vi "Registers.vi"(0 "register instruction":T6, 5 "config.resources":T4, 7 "sync.resources":T7, 9 "time.resources":T3) -> (4 "read completion out":T5, 14 "ready for input":bool)   [LabVIEW 2023]
uses:
  <instrlib>/niUSRPRIO/GPS/v1/FPGA/niUsrpRio GPS v1 FPGA.lvlib
  <instrlib>/niUsrpRio/Config/v1/FPGA/niUsrpRio Config v1 FPGA.lvlib
  <instrlib>/niUSRPRIO/Time/v1/FPGA/niUsrpRio Time v1 FPGA.lvlib
  <instrlib>/niUSRPRIO/Synchronization/v1/FPGA/niUsrpRio Synchronization v1 FPGA.lvlib
  <instrlib>/_niInstr/Register Bus/v1/FPGA/Private/Mux/Read Completion Mux (6 inputs).vi
  <instrlib>/niUSRPRIO/Synchronization/v1/FPGA/Private/Resources.ctl
  <instrlib>/_niInstr/Register Bus/v1/FPGA/Public/Register Instruction.ctl
  <instrlib>/niUSRPRIO/Time/v1/FPGA/Private/Future Event Resources.ctl
  <instrlib>/niUSRPRIO/Time/v1/FPGA/Private/Time Resources.ctl
  <instrlib>/_niInstr/Register Bus/v1/FPGA/Public/Read Completion.ctl
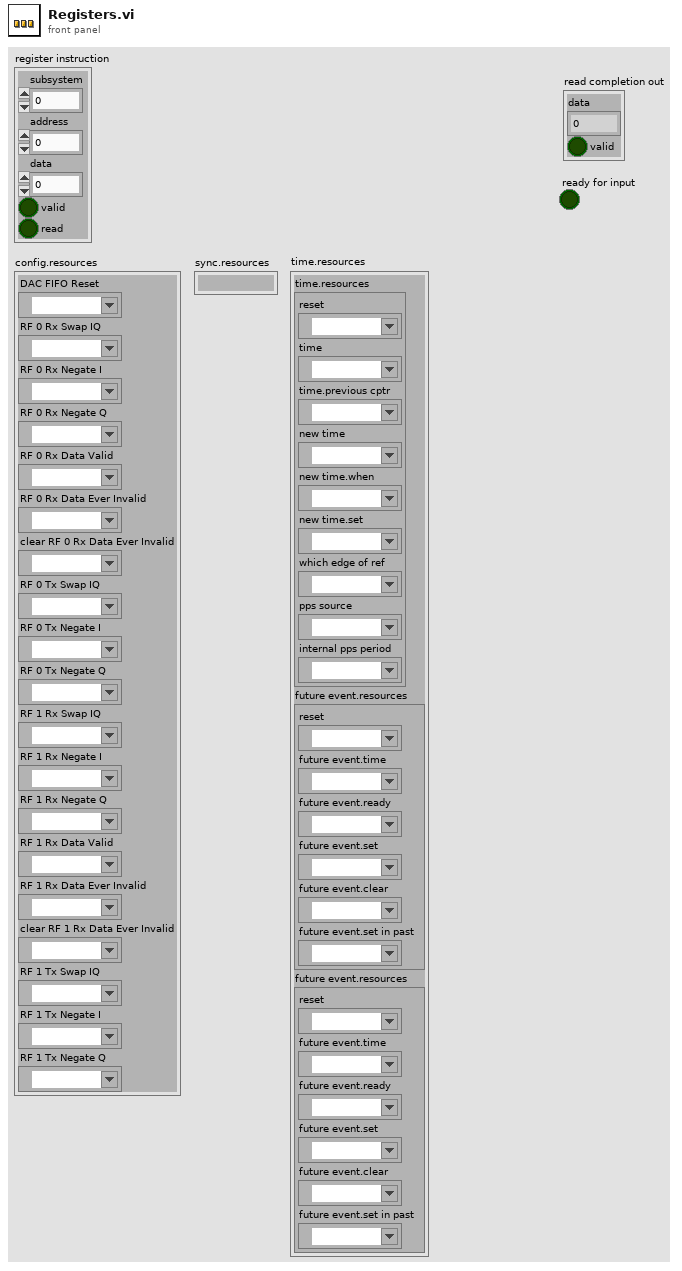
[diagram p1: front panel]
types:
  T1 = typedef "niUsrpRio Time v1 FPGA.lvlib/Time Resources.ctl" = cluster{"reset":refnum<k21>, "time":refnum<k21>, "time.previous cptr":refnum<k21>, "new time":refnum<k21>, "new time.when":refnum<k21>, "new time.set":refnum<k21>, "which edge of ref":refnum<k21>, "pps source":refnum<k21>, "internal pps period":refnum<k21>}
  T2 = typedef "niUsrpRio Time v1 FPGA.lvlib/Future Event Resources.ctl" = cluster{"reset":refnum<k21>, "future event.time":refnum<k21>, "future event.ready":refnum<k21>, "future event.set":refnum<k21>, "future event.clear":refnum<k21>, "future event.set in past":refnum<k21>}
  T3 = cluster{"time.resources":T1, "future event.resources":T2, "future event.resources":T2}
  T4 = cluster{"DAC FIFO Reset":refnum<k21>, "RF 0 Rx Swap IQ":refnum<k21>, "RF 0 Rx Negate I":refnum<k21>, "RF 0 Rx Negate Q":refnum<k21>, "RF 0 Rx Data Valid":refnum<k21>, "RF 0 Rx Data Ever Invalid":refnum<k21>, "clear RF 0 Rx Data Ever Invalid":refnum<k21>, "RF 0 Tx Swap IQ":refnum<k21>, "RF 0 Tx Negate I":refnum<k21>, "RF 0 Tx Negate Q":refnum<k21>, "RF 1 Rx Swap IQ":refnum<k21>, "RF 1 Rx Negate I":refnum<k21>, "RF 1 Rx Negate Q":refnum<k21>, "RF 1 Rx Data Valid":refnum<k21>, "RF 1 Rx Data Ever Invalid":refnum<k21>, "clear RF 1 Rx Data Ever Invalid":refnum<k21>, "RF 1 Tx Swap IQ":refnum<k21>, "RF 1 Tx Negate I":refnum<k21>, "RF 1 Tx Negate Q":refnum<k21>}
  T5 = typedef "niInstr Register Bus v1 FPGA.lvlib/Read Completion.ctl" = cluster{"data":u32, "valid":bool}
  T6 = typedef "niInstr Register Bus v1 FPGA.lvlib/Register Instruction.ctl" = cluster{"subsystem":u8, "address":u16, "data":u32, "valid":bool, "read":bool}
  T7 = typedef "niUsrpRio Synchronization v1 FPGA.lvlib/Resources.ctl" = cluster{"master":refnum<k21>, "meas.enable":refnum<k21>, "meas.ready":refnum<k21>, "meas.reset":refnum<k21>, "meas.arm":refnum<k21>, "meas.valid":refnum<k21>, "meas.value":refnum<k21>, "meas.oversample factor":refnum<k21>, "cptr":refnum<k21>, "cptr.adjust":refnum<k21>, "cptr.period":refnum<k21>}
  T8 = enum8{"rx.start trigger event", "tx.start trigger event"}
  T9 = cluster{"read completion":T5, "read completion":T5}
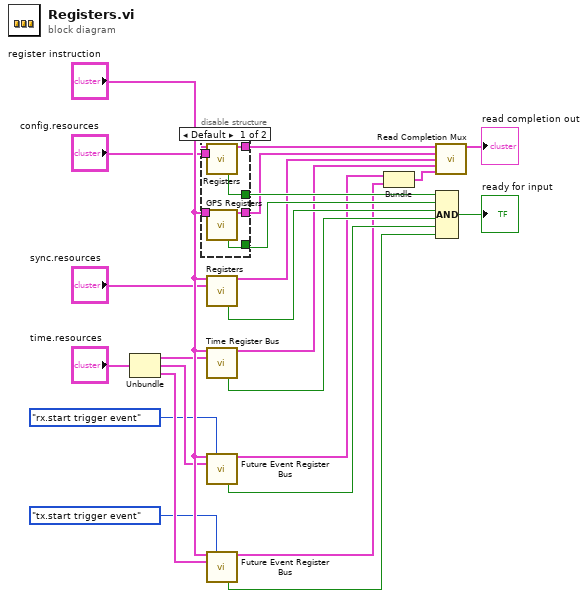
[diagram p0: block diagram]
diagram:
  n1 = Unbundle("time.resources") -> ("time.resources"=w5:T1, "future event.resources"=w4:T2, "future event.resources"=w3:T2)
  n2 = disable-structure shown="Default" {
    disable-tunnel: [w30 _] -> w20
    disable-tunnel: [w29 _] -> w19
    disable-tunnel: "register instruction" -> [w28 _]
    disable-tunnel: [w27 _] -> w11
    disable-tunnel: [w26 _] -> w10
    disable-tunnel: "config.resources" -> [w25 _]
    frame condition #0 (active) {
      n3 = call <instrlib>:"Registers.vi"("register instruction"=w28, "resources"=w25) -> ("read completion out"=w26:T5, "ready for input"=w29:bool)  [unwired: 12 in]
      n4 = call <instrlib>:"GPS Registers.vi"("register instruction"=w28) -> ("read completion"=w27:T5, "ready for input"=w30:bool)  [unwired: 13 in]
    }
    frame condition #1 {
    }
  }
  n5 = call <instrlib>:"Registers.vi"("register instruction"="register instruction", "sync.resources"="sync.resources") -> ("read completion"=w16:T5, "ready for input"=w21:bool)  [unwired: 12 in]
  n6 = call <instrlib>:"Time Register Bus.vi"("register instruction"="register instruction", "time.resources"=w5) -> ("read completion"=w15:T5, "ready for input"=w22:bool)  [unwired: 12 in]
  n7 = call <instrlib>:"Future Event Register Bus.vi"("register instruction"="register instruction", "instance"=T8."rx.start trigger event", "future event.resources"=w4) -> ("read completion"=w13:T5, "ready for input"=w23:bool)  [unwired: 11 in]
  n8 = call <instrlib>:"Future Event Register Bus.vi"("register instruction"="register instruction", "instance"=T8."tx.start trigger event", "future event.resources"=w3) -> ("read completion"=w12:T5, "ready for input"=w24:bool)  [unwired: 11 in]
  n9 = Bundle("read completion"=w13, "read completion"=w12) -> (w14:T9)  [unwired: 1 in]
  n10 = call-poly <instrlib>:"Read Completion Mux.vi"("element 0"=w10, "element 1"=w11, "element 2"=w16, "element 3"=w15, "remaining elements (cluster)"=w14) -> ("read completion out"=→"read completion out":T5)  [unwired: 10 in]
  n11 = Compound Arithmetic op=AND(w19, w20, w21, w22, w23, w24) -> (→"ready for input":bool)
